vi "PH_AWG-510.Pack Output Settings.vi"(0 "Activate Channel":bool, 1 "VPP [Volts]":dbl, 3 "Clock [Hz]":dbl, 4 "File Name":string, 5 "Waveform Pattern [#1 ... #20]":u16[](array[numeric])) -> (17 "Output Settings":T1={"Activate Channel"=FALSE, "VPP (V)"=0.0, "Clock (Hz)"=0.0, "File Name (Device)"="", "#1"=0, "#2"=0, "#3"=0, "#4"=0, "#5"=0, "#6"=0, "#7"=0, "#8"=0, "#9"=0, "#10"=0, "#11"=0, "#12"=0, "#13"=0, "#14"=0, "#15"=0, "#16"=0, "#17"=0, "#18"=0, "#19"=0, "#20"=0, "Offset (V)"=-1.0} {"#20" max=1023 step=1 scale=0.0..1023.0; "#19" max=1023 step=1 scale=0.0..1023.0; "#18" max=1023 step=1 scale=0.0..1023.0; "#17" max=1023 step=1 scale=0.0..1023.0; "#16" max=1023 step=1 scale=0.0..1023.0; "#15" max=1023 step=1 scale=0.0..1023.0; "#14" max=1023 step=1 scale=0.0..1023.0; "#13" max=1023 step=1 scale=0.0..1023.0; "#12" max=1023 step=1 scale=0.0..1023.0; "#11" max=1023 step=1 scale=0.0..1023.0; "#10" max=1023 step=1 scale=0.0..1023.0; "#9" max=1023 step=1 scale=0.0..1023.0; "#8" max=1023 step=1 scale=0.0..1023.0; "#7" max=1023 step=1 scale=0.0..1023.0; "#6" max=1023 step=1 scale=0.0..1023.0; "#5" max=1023 step=1 scale=0.0..1023.0; "#4" max=1023 step=1 scale=0.0..1023.0; "#3" max=1023 step=1 scale=0.0..1023.0; "#2" max=1023 step=1 scale=0.0..1023.0; "#1" max=1023 step=1 scale=0.0..1023.0})   [LabVIEW 2014, in "PH_AWG-510.lvlib"]
uses:
  PH_AWG-510.lvlib
  PH_AWG-510.Output Settings.ctl
panel:
  # "Waveform Pattern"
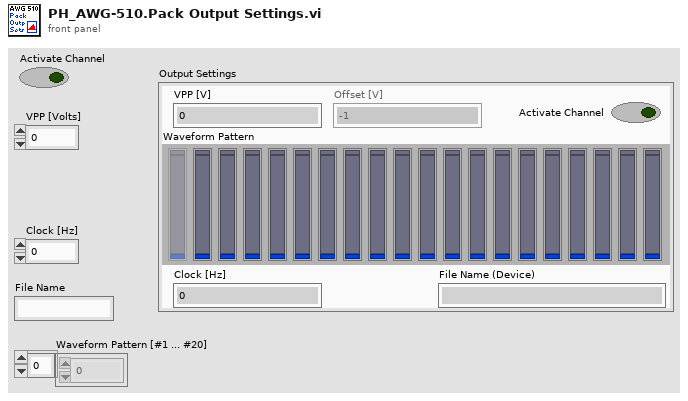
[diagram p1: front panel]
types:
  T1 = typedef "PH_AWG-510.lvlib/PH_AWG-510.Output Settings.ctl" = cluster{"Activate Channel":bool, "VPP (V)":dbl, "Clock (Hz)":dbl, "File Name (Device)":string, "#1":u16, "#2":u16, "#3":u16, "#4":u16, "#5":u16, "#6":u16, "#7":u16, "#8":u16, "#9":u16, "#10":u16, "#11":u16, "#12":u16, "#13":u16, "#14":u16, "#15":u16, "#16":u16, "#17":u16, "#18":u16, "#19":u16, "#20":u16, "Offset (V)":dbl}
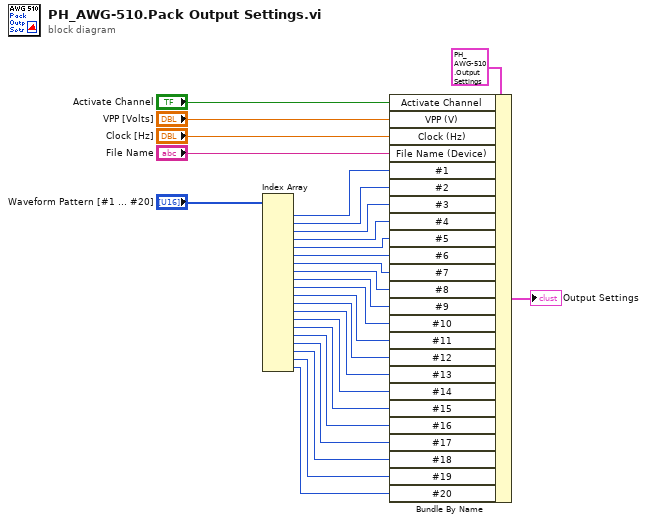
[diagram p0: block diagram]
diagram:
  n1 = Index Array(array="Waveform Pattern [#1 ... #20]") -> (element #1=w1:u16, element #2=w26:u16, element #3=w27:u16, element #4=w9:u16, element #5=w10:u16, element #6=w11:u16, element #7=w12:u16, element #8=w13:u16, element #9=w14:u16, element #10=w15:u16, element #11=w16:u16, element #12=w17:u16, element #13=w18:u16, element #14=w19:u16, element #15=w20:u16, element #16=w21:u16, element #17=w22:u16, element #18=w23:u16, element #19=w24:u16, element #20=w25:u16)  [unwired: 20 in]
  n2 = Bundle By Name(cluster=T1 {"Activate Channel"=FALSE, "VPP (V)"=0.0, "Clock (Hz)"=0.0, "File Name (Device)"="", "#1"=0, "#2"=0, "#3"=0, "#4"=0, "#5"=0, "#6"=0, "#7"=0, "#8"=0, "#9"=0, "#10"=0, "#11"=0, "#12"=0, "#13"=0, "#14"=0, "#15"=0, "#16"=0, "#17"=0, "#18"=0, "#19"=0, "#20"=0, "Offset (V)"=-1.0} ("Wanted Trigger Settings"), "Activate Channel"="Activate Channel", "VPP (V)"="VPP [Volts]", "Clock (Hz)"="Clock [Hz]", "File Name (Device)"="File Name", "#1"=w1, "#2"=w26, "#3"=w27, "#4"=w9, "#5"=w10, "#6"=w11, "#7"=w12, "#8"=w13, "#9"=w14, "#10"=w15, "#11"=w16, "#12"=w17, "#13"=w18, "#14"=w19, "#15"=w20, "#16"=w21, "#17"=w22, "#18"=w23, "#19"=w24, "#20"=w25) -> (→"Output Settings":T1)
